vi "vipm_BuildDailyVIP.vi"(8 "error in (no error)":errorcluster, 11 "CommandLine":string[](array[string])) -> (0 "error out":errorcluster, 2 "test details":string, 3 "output to action":string)   [LabVIEW 2014]
uses:
  <userlib>/_OpenG.lib/file/file.llb/File Exists - Scalar__ogtk.vi
  <userlib>/_OpenG.lib/string/string.llb/Trim Whitespace (String)__ogtk.vi
  <vilib>/JKI/VIPM API/VIPM API_vipm_api.lvlib
  _lvcicd/_lvcicd_support_2014.lvlib
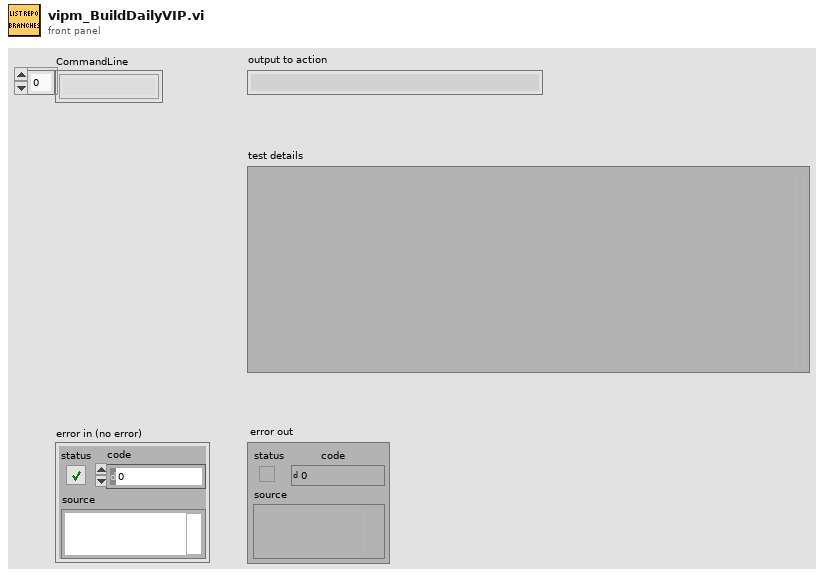
[diagram p1: front panel]
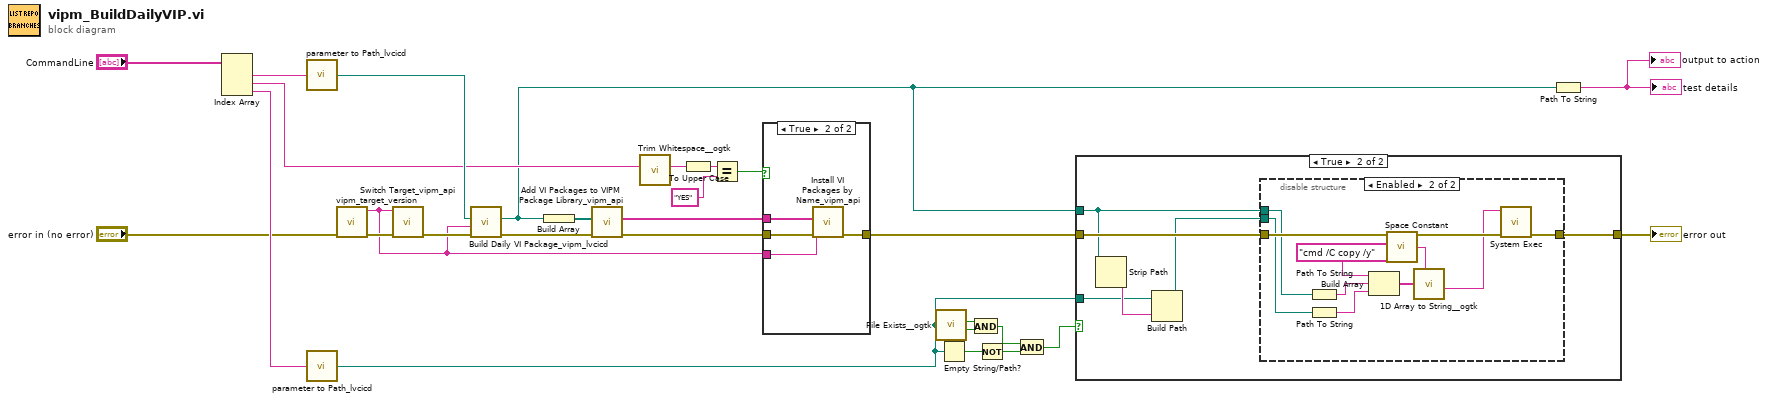
[diagram p0: block diagram]
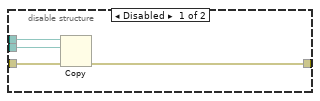
[diagram p3: hidden frame]
diagram:
  n1 = Index Array(array="CommandLine") -> (element #1=w25:string, element #2=w18:string, element #3=w13:string)  [unwired: 3 in]
  n2 = call "parameter to Path_lvcicd.vi"("String"=w25) -> ("Path"=w27:path)
  n3 = call "parameter to Path_lvcicd.vi"("String"=w13) -> ("Path"=w14:path)
  n4 = call "vipm_target_version.vi"() -> ("vipm Taget version"=w2:string)  [unwired: 11 in]
  n5 = call <vilib>:"Switch Target_vipm_api.vi"("error in (no error)"="error in (no error)", "LabVIEW Version"=w2) -> ("error out"=w3:errorcluster)  [unwired: 9 in]
  n6 = call "Build Daily VI Package_vipm_lvcicd.vi"("error in (no error)"=w3, "LabVIEW Version"=w2, "vipb"=w27) -> ("error out"=w23:errorcluster, "Build Output"=w11:path)  [unwired: 5 in, 2 out]
  n7 = Build Array(w11) -> (w24:path[])
  n8 = call <vilib>:"Add VI Packages to VIPM Package Library_vipm_api.vi"("error in (no error)"=w23, "Packages to add to VIPM Library (vipc,vip,ogp)"=w24) -> ("error out"=w22:errorcluster, "Package Names Added"=w21:string[])  [unwired: 8 in]
  n9 = call-poly <userlib>:"Trim Whitespace__ogtk.vi"("String in"=w18) -> ("String out"=w15:string)  [unwired: 6 in]
  n10 = To Upper Case(1:w15) -> (0:w16:string)
  n11 = Equal?(x=w16, y="YES") -> (x = y?=w19:bool)
  n12 = case shown="True" w19 {
    tunnel: w22 -> [w28 w32]
    tunnel: [w28 w31] -> w20
    tunnel: w2 -> [_ w30]
    tunnel: w21 -> [_ w29]
    frame False {
    }
    frame True {
      n13 = call <vilib>:"Install VI Packages by Name_vipm_api.vi"("error in (no error)"=w32, "LabVIEW Version"=w30, "Package Names to Install []"=w29) -> ("error out"=w31:errorcluster)  [unwired: 8 in]
    }
  }
  n14 = call-poly <userlib>:"File Exists__ogtk.vi"("file path"=w14) -> ("is directory"=w10:bool, "exists"=w9:bool)  [unwired: 6 in]
  n15 = Empty String/Path?(string/path=w14) -> (empty?=w8:bool)
  n16 = And(x=w10, y=w9) -> (x .and. y?=w7:bool)
  n17 = Not(x=w8) -> (.not. x?=w5:bool)
  n18 = And(x=w7, y=w5) -> (x .and. y?=w6:bool)
  n19 = case shown="True" w6 {
    tunnel: w20 -> [w33 w39]
    tunnel: [w33 w38] -> w12
    tunnel: w11 -> [_ w36]
    tunnel: w14 -> [_ w34]
    frame False {
    }
    frame True {
      n20 = Strip Path(path=w36) -> (name=w35:string)  [unwired: 1 out]
      n21 = Build Path(base path=w34, name or relative path=w35) -> (appended path=w37:path)
      n22 = disable-structure shown="Enabled" {
        disable-tunnel: w39 -> [w43 w52]
        disable-tunnel: [w42 w53] -> w38
        disable-tunnel: w37 -> [w41 w50]
        disable-tunnel: w36 -> [w40 w51]
        frame Disabled {
          n23 = Copy(8:w43, 10:w41, 11:w40) -> (0:w42:errorcluster)  [unwired: 2 in, 2 out]
        }
        frame Enabled {
          n24 = Path To String(path=w51) -> (string=w48:string)
          n25 = Path To String(path=w50) -> (string=w47:string)
          n26 = Build Array("cmd /C copy /y" ("name"), w48, w47) -> (w46:string[])
          n27 = call <vilib>:"Space Constant.vi"() -> ("String"=w45:string)
          n28 = call <userlib>:"1D Array to String__ogtk.vi"("delimiter (Tab)"=w45, "Array of Strings"=w46) -> ("delimited string"=w44:string)  [unwired: 9 in]
          n29 = call <vilib>:"System Exec.vi"("error in (no error)"=w52, "command line"=w44) -> ("error out"=w53:errorcluster)  [unwired: 6 in, 3 out]
        }
      }
    }
  }
  "error out" <- w12
  n30 = Path To String(path=w11) -> (string=→"test details" →"output to action":string)
